vi "Change String.vi"(8 "AutoComplete?":bool, 9 "Match Cluster":cluster{"Item Index":i32, "Offset":i32}, 10 "Keyword Array":string[](array[string]), 11 "String Refnum":refnum<vi>) -> (3 "String Value":string)   [LabVIEW 2011, in "Intellisense Xcontrol.xctl"]
uses:
  Intellisense Xcontrol.xctl
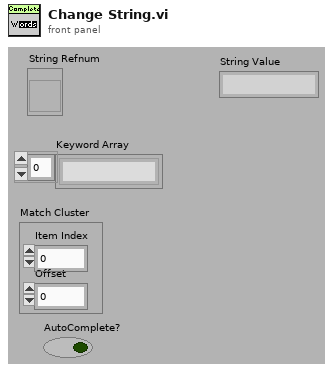
[diagram p1: front panel]
types:
  T1 = cluster{"Selection Start":u32, "Selection End":u32}
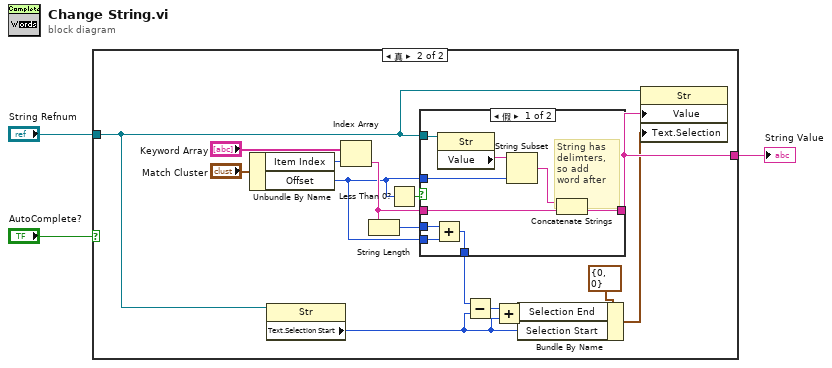
[diagram p0: block diagram]
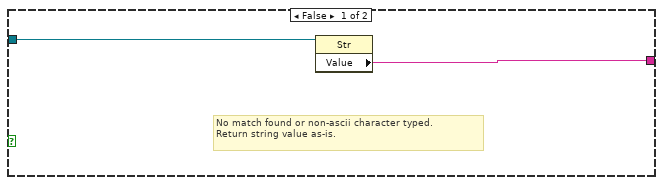
[diagram p2: hidden frame]
diagram:
  n1 = case shown="真" "AutoComplete?" {
    tunnel: [w4 w13] -> w3
    tunnel: "String Refnum" -> [w5 w6]
    frame False {
      # "No match found or non-ascii character typed.\nReturn string value as-is."
      n2 = property class="Str"(reference=w5) -> ("Value"=w4:string)  [unwired: 1 in, 2 out]
    }
    frame True {
      n3 = Unbundle By Name("Match Cluster") -> ("Item Index"=w14:i32, "Offset"=w8:i32)
      n4 = property on="Property Node" class="Str"(reference=w6) -> ("Text.Selection Start"=w16:u32)  [unwired: 1 in, 2 out]
      n5 = Index Array(array="Keyword Array", index=w14) -> (element=w12:string)
      n6 = String Length(string=w12) -> (length=w10:i32)
      n7 = Less Than 0?(x=w8) -> (x < 0?=w11:bool)
      n8 = case shown="假" w11 {
        tunnel: [w27 w31] -> w13
        tunnel: w12 -> [w26 w31]
        tunnel: w8 -> [w25 _]
        tunnel: w10 -> [w23 w30]
        tunnel: [w22 w30] -> w9
        tunnel: w8 -> [w24 _]
        tunnel: w6 -> [w21 _]
        frame False {
          # "String has\ndelimters,\nso add\nword after"
          n9 = Add(x=w23, y=w24) -> (x+y=w22:i32)
          n10 = property class="Str"(reference=w21) -> ("Value"=w29:string)  [unwired: 1 in, 2 out]
          n11 = String Subset(string=w29, length (rest)=w25) -> (substring=w28:string)  [unwired: 1 in]
          n12 = Concatenate Strings(w28, w26) -> (w27:string)
        }
        frame True {
          # "String has no spaces,\nreplace entire word"
        }
      }
      n13 = Subtract(x=w9, y=w16) -> (x-y=w17:u32)
      n14 = Add(x=w17, y=w16) -> (x+y=w15:u32)
      n15 = Bundle By Name(cluster=T1 {"Selection Start"=0, "Selection End"=0} ("Text.Selection"), "Selection End"=w15, "Selection Start"=w16) -> (w7:T1)
      n16 = property on="Property Node" class="Str"(reference=w6, "Value"=w13, "Text.Selection"=w7) -> ()  [unwired: 1 in, 2 out]
    }
  }
  "String Value" <- w3
